vi "ANNsubs_NormalizedAngular.vi"(1 "Delta angle":dbl) -> (0 "Delta angle out":dbl)   [LabVIEW 2017]
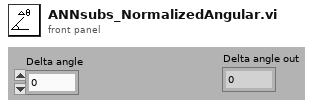
[diagram p1: front panel]
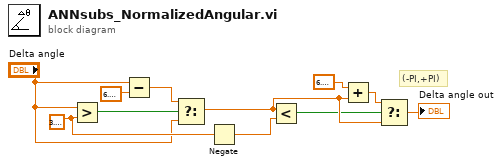
[diagram p0: block diagram]
diagram:
  w5 = 3.141592653589793
  # "(-PI,+PI)"
  n1 = Greater?(x="Delta angle", y=w5) -> (0:w2:bool)
  n2 = Subtract(x="Delta angle", y=6.283185307179586) -> (x-y=w3:dbl)
  n3 = Select(t=w3, s=w2, f="Delta angle") -> (s? t:f=w10:dbl)
  n4 = Negate(x=w5) -> (-x=w6:dbl)
  n5 = Less?(x=w10, y=w6) -> (x < y?=w9:bool)
  n6 = Add(x=6.283185307179586, y=w10) -> (x+y=w8:dbl)
  n7 = Select(t=w8, s=w9, f=w10) -> (s? t:f=→"Delta angle out":dbl)
